vi "任意波形绘制.vi"(8 "曲线设置":T2, 10 "历史数据":cluster{"数据":dbl[][]}[](array[cluster]), 11 "映射方式":T1) -> (0 "曲线属性":cluster{"曲线名":string, "曲线颜色":u32, "线条宽度":u8}[](array[cluster]), 3 "XY图":cluster{"数据":dbl[], "数据":dbl[]}[](array[cluster]))   [LabVIEW 2020, in "数据显示.xctl"]
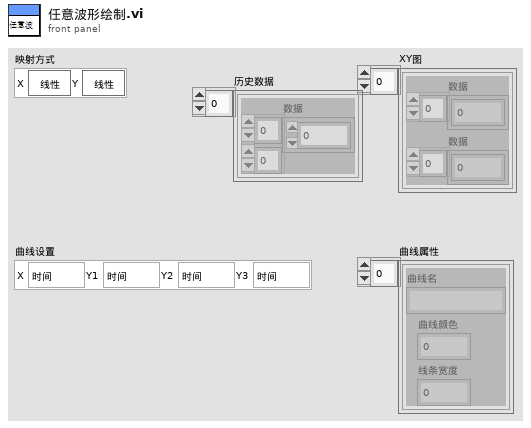
[diagram p1: front panel]
types:
  T1 = typedef "数据显示.xctl/映射方式.ctl" = cluster{"X":bool, "Y":bool}
  T2 = typedef "数据显示.xctl/曲线设置.ctl" = cluster{"X":enum16{"时间", "设置电压", "读取电流", "读取电压"}, "Y1":enum16{"时间", "设置电压", "读取电流", "读取电压"}, "Y2":enum16{"时间", "设置电压", "读取电流", "读取电压", "无"}, "Y3":enum16{"时间", "设置电压", "读取电流", "读取电压", "无"}}
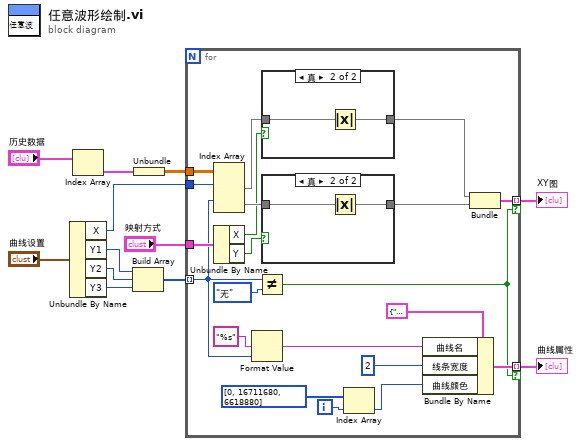
[diagram p0: block diagram]
diagram:
  n1 = Unbundle By Name("曲线设置") -> ("X"=w3:enum16{"时间", "设置电压", "读取电流", "读取电压"}, "Y1"=w4:enum16{"时间", "设置电压", "读取电流", "读取电压"}, "Y2"=w5:enum16{"时间", "设置电压", "读取电流", "读取电压", "无"}, "Y3"=w6:enum16{"时间", "设置电压", "读取电流", "读取电压", "无"})
  n2 = Index Array(array="历史数据") -> (element=w9:cluster{"数据":dbl[][]})  [unwired: 1 in]
  n3 = Build Array(w4, w5, w6) -> (w7:enum16{"时间", "设置电压", "读取电流", "读取电压", "无"}[])
  n4 = Unbundle(w9) -> ("数据"=w10:dbl[][])
  n5 = for {
    tunnel: w10 -> [w33]
    tunnel: w3 -> [w32]
    tunnel: w7 -> [w15] mode=indexing
    tunnel: "映射方式" -> [w31]
    tunnel: [w23] -> w12 mode=indexing if=w19
    tunnel: [w22] -> w11 mode=indexing if=w19
    i -> [w17]
    n6 = Index Array(array=w33, index (row) #1=w32, index (row) #2=w15) -> (element #1=w30:dbl[], element #2=w29:dbl[])  [unwired: 2 in]
    n7 = Unbundle By Name(w31) -> ("X"=w26:bool, "Y"=w25:bool)
    n8 = Format Value(format string="%s" ("格式字符串"), value (0)=w15) -> (output string=w13:string)  [unwired: 1 in]
    n9 = Not Equal?(x=w15, y=enum16{"时间", "设置电压", "读取电流", "读取电压", "无"}."无") -> (x != y?=w19:bool)
    n10 = case shown="真" w26 {
      tunnel: w30 -> [w37 w39]
      tunnel: [w37 w38] -> w28
      frame False {
      }
      frame True {
        n11 = Absolute Value(x=w39) -> (abs(x)=w38:dbl[])
      }
    }
    n12 = case shown="真" w25 {
      tunnel: w29 -> [w34 w36]
      tunnel: [w34 w35] -> w27
      frame False {
      }
      frame True {
        n13 = Absolute Value(x=w36) -> (abs(x)=w35:dbl[])
      }
    }
    n14 = Index Array(array=u32[] [0, 16711680, 6618880], index=w17) -> (element=w16:u32)
    n15 = Bundle By Name(cluster=cluster{"曲线名":string, "曲线颜色":u32, "线条宽度":u8} {"曲线名"="", "曲线颜色"=0, "线条宽度"=0} ("曲线属性"), "曲线名"=w13, "线条宽度"=u8 2, "曲线颜色"=w16) -> (w22:cluster{"曲线名":string, "曲线颜色":u32, "线条宽度":u8})
    n16 = Bundle("数据"=w28, "数据"=w27) -> (w23:cluster{"数据":dbl[], "数据":dbl[]})  [unwired: 1 in]
  }
  "XY图" <- w12
  "曲线属性" <- w11
